vi "Initialize.vi"(8 "error in (no error)":errorcluster, 11 "Channel in":refnum<class "Channel.lvclass">) -> (0 "error out":errorcluster, 3 "Channel out":refnum<class "Channel.lvclass">)   [LabVIEW 2018, in "Channel.lvclass"]
uses:
  Channel.lvclass
  StateMachine/State Machine.lvclass
  Interface/Interface.lvclass
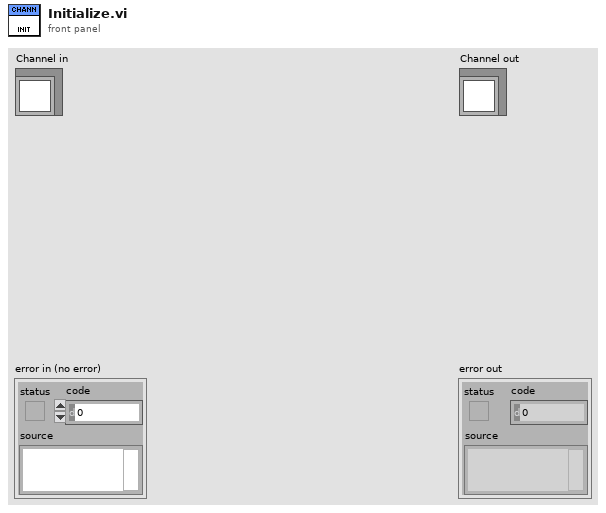
[diagram p1: front panel]
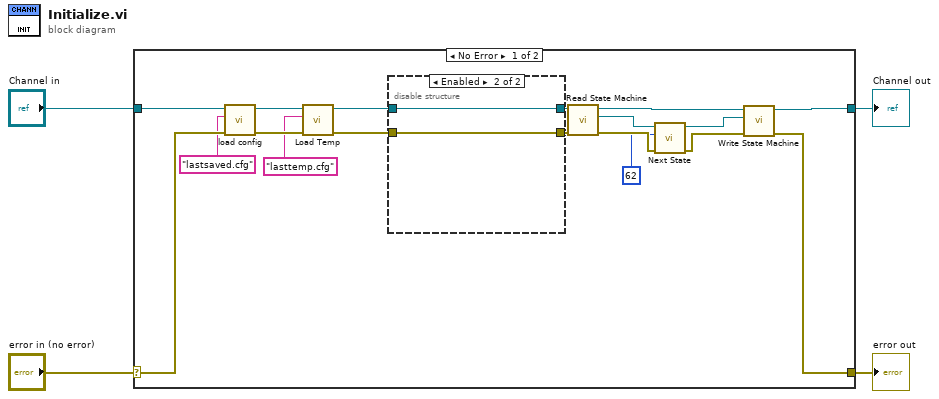
[diagram p0: block diagram]
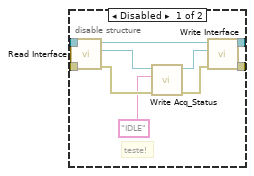
[diagram p2: hidden frame]
diagram:
  n1 = case shown="No Error" "error in (no error)" {
    selector: "error in (no error)" -> [w13 w36]
    tunnel: [w16 w36] -> w3
    tunnel: [w17 w35] -> w1
    tunnel: "Channel in" -> [w14 w35]
    frame No Error {
      n2 = call-dynamic "load config.vi"("error in (no error)"=w13, "cfg file name"="lastsaved.cfg", "Channel in"=w14) -> ("error out"=w7:errorcluster, "Channel out"=w9:refnum<class "Channel.lvclass">)  [unwired: 7 in]
      n3 = call-dynamic "Load Temp.vi"("error in (no error)"=w7, "temp file name"="lasttemp.cfg", "Channel in"=w9) -> ("error out"=w6:errorcluster, "Channel out"=w8:refnum<class "Channel.lvclass">)  [unwired: 7 in]
      n4 = disable-structure shown="Enabled" {
        disable-tunnel: w8 -> [w32 w34]
        disable-tunnel: [w30 w34] -> w11
        disable-tunnel: w6 -> [w27 w33]
        disable-tunnel: [w24 w33] -> w10
        frame Disabled {
          # "teste!"
          n5 = call-dynamic "Read Interface.vi"("error in (no error)"=w27, "Channel in"=w32) -> ("error out"=w26:errorcluster, "Interface.lvclass"=w29:refnum<class "Interface.lvclass">, "Channel out"=w31:refnum<class "Channel.lvclass">)  [unwired: 7 in]
          n6 = call-dynamic "Write Acq_Status.vi"("error in (no error)"=w26, "Acq_Status"="IDLE", "Interface in"=w29) -> ("error out"=w25:errorcluster, "Interface out"=w28:refnum<class "Interface.lvclass">)  [unwired: 7 in]
          n7 = call-dynamic "Write Interface.vi"("error in (no error)"=w25, "Interface.lvclass"=w28, "Channel in"=w31) -> ("error out"=w24:errorcluster, "Channel out"=w30:refnum<class "Channel.lvclass">)  [unwired: 7 in]
        }
        frame Enabled {
        }
      }
      n8 = call-dynamic "Read State Machine.vi"("error in (no error)"=w10, "Device in"=w11) -> ("error out"=w21:errorcluster, "State Machine.lvclass"=w22:refnum<class "State Machine.lvclass">, "Device out"=w18:refnum<class "Channel.lvclass">)  [unwired: 7 in]
      n9 = call "Next State.vi"("error in (no error)"=w21, "New_State"=62, "State Machine in"=w22) -> ("error out"=w19:errorcluster, "State Machine out"=w20:refnum<class "State Machine.lvclass">)  [unwired: 7 in]
      n10 = call-dynamic "Write State Machine.vi"("error in (no error)"=w19, "State Machine.lvclass"=w20, "Device in"=w18) -> ("error out"=w16:errorcluster, "Device out"=w17:refnum<class "Channel.lvclass">)  [unwired: 7 in]
    }
    frame Error {
    }
  }
  "error out" <- w3
  "Channel out" <- w1
